vi "Get Size.vi"(11 "Pointer in":refnum<class "Pointer.lvclass">) -> (2 "size":u64 format="%d bytes", 3 "Pointer out":refnum<class "Pointer.lvclass">)   [LabVIEW 2027, in "Memory Manager.lvlib" / "Pointer.lvclass"]
uses:
  Pointer.lvclass
  Pointer.lvclass/Pointer.ctl
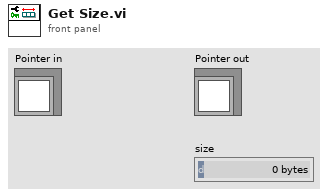
[diagram p1: front panel]
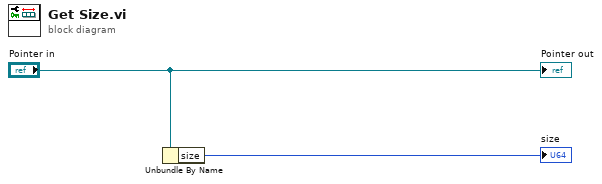
[diagram p0: block diagram]
diagram:
  n1 = Unbundle By Name("Pointer in") -> ("size"=→"size":u64)
  "Pointer out" <- "Pointer in"
